vi "UV-VIS CoolerOFF.vi"(3 "error in (no error)":errorcluster, 5 "UV-VIS  in":refnum<class "CCD_camera.lvclass">) -> (0 "error out":errorcluster, 1 "DLL error code":u32, 2 "UV-VIS  out":refnum<class "CCD_camera.lvclass">)   [LabVIEW 2020, in "CCD_camera.lvclass"]
doc: "Switches OFF the cooling. The rate of temperature change is controlled until the temperature reaches 0 degrees. Control is returned immediately to the calling application.\n\n<B>Error codes:</B>\nDRV_SUCCESS - Temperature controller switched OFF.\nDRV_NOT_INITIALIZED - System not initialized.\nDRV_ACQUIRING - Acquisition in progress.\nDRV_ERROR_ACK - Unable to communicate with card.\n\n<B>NOTES:</B>\n<B>When the temperature control is switched OFF the temperature of the sensor is gradually raised to zero degrees to ensure no thermal stresses are set up in the sensor. When closing down the program via ShutDown you must ensure that the temperature of the detector is above zero degrees. Otherwise calling ShutDown while the detector is still cooled will cause the temperature to raise faster than certified.</B>"
uses:
  CCD_camera.lvclass
  C:/dev/TRANCON/Classes/Detector/Detector.lvclass
  Detector.lvclass/Detector.ctl
  Detector.lvclass
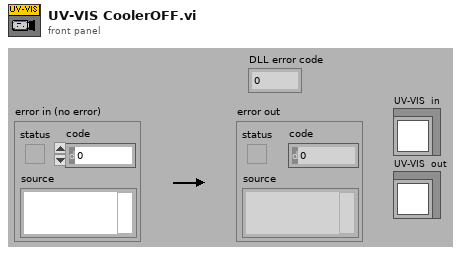
[diagram p1: front panel]
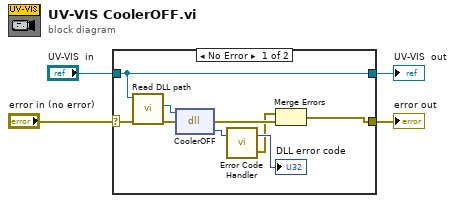
[diagram p0: block diagram]
diagram:
  n1 = case shown="No Error" "error in (no error)" {
    selector: "error in (no error)" -> [w10 w15]
    tunnel: [w6 w15] -> w3
    tunnel: [w11 w14] -> w2
    tunnel: "UV-VIS  in" -> [w11 w14]
    frame No Error {
      n2 = call "Read DLL path.vi"("error in (no error)"=w10, "Detector in"=w11) -> ("error out"=w9:errorcluster, "DLL path"=w5:path)  [unwired: 7 in, 1 out]
      n3 = dll-call lib="S:/TRANCON/DLL/Atmcd32d.dll" fn="CoolerOFF"(path in=w5, error in=w9) -> (error out=w8:errorcluster, "return type"=w13:u32)  [unwired: 1 in, 1 out]
      n4 = call "Error Code Handler.vi"("DLL error code"=w13) -> ("error out"=w7:errorcluster, "dup DLL error code"=→"DLL error code":u32)  [unwired: 1 in]
      n5 = Merge Errors(w7, w8) -> (w6:errorcluster)
    }
    frame Error {
    }
  }
  "error out" <- w3
  "UV-VIS  out" <- w2
